vi "synchronization_0.vi"(11 "sweep signal":dbl[](array[numeric])=array[10000 elements]) -> (0 "Micro 1/ ai 2":dbl[](graph), 3 "Micro 2/ai 1":dbl[](graph))   [LabVIEW 2014]
uses:
  <vilib>/DAQmx/configure/timing.llb/DAQmx Timing (Sample Clock).vi
  <vilib>/DAQmx/create/channels.llb/DAQmx Create Channel (AO-Voltage-Basic).vi
  <vilib>/DAQmx/write.llb/DAQmx Write (Analog 1D DBL 1Chan NSamp).vi
  <vilib>/DAQmx/create/channels.llb/DAQmx Create Channel (AI-Voltage-Basic).vi
  <vilib>/DAQmx/read.llb/DAQmx Read (Analog 2D DBL NChan NSamp).vi
panel:
  out "Sweep":dbl[](graph)
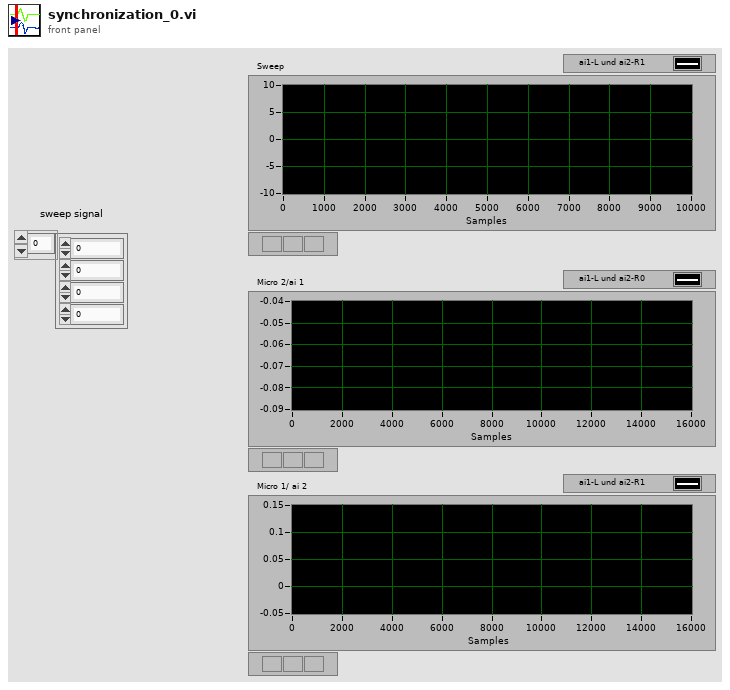
[diagram p1: front panel]
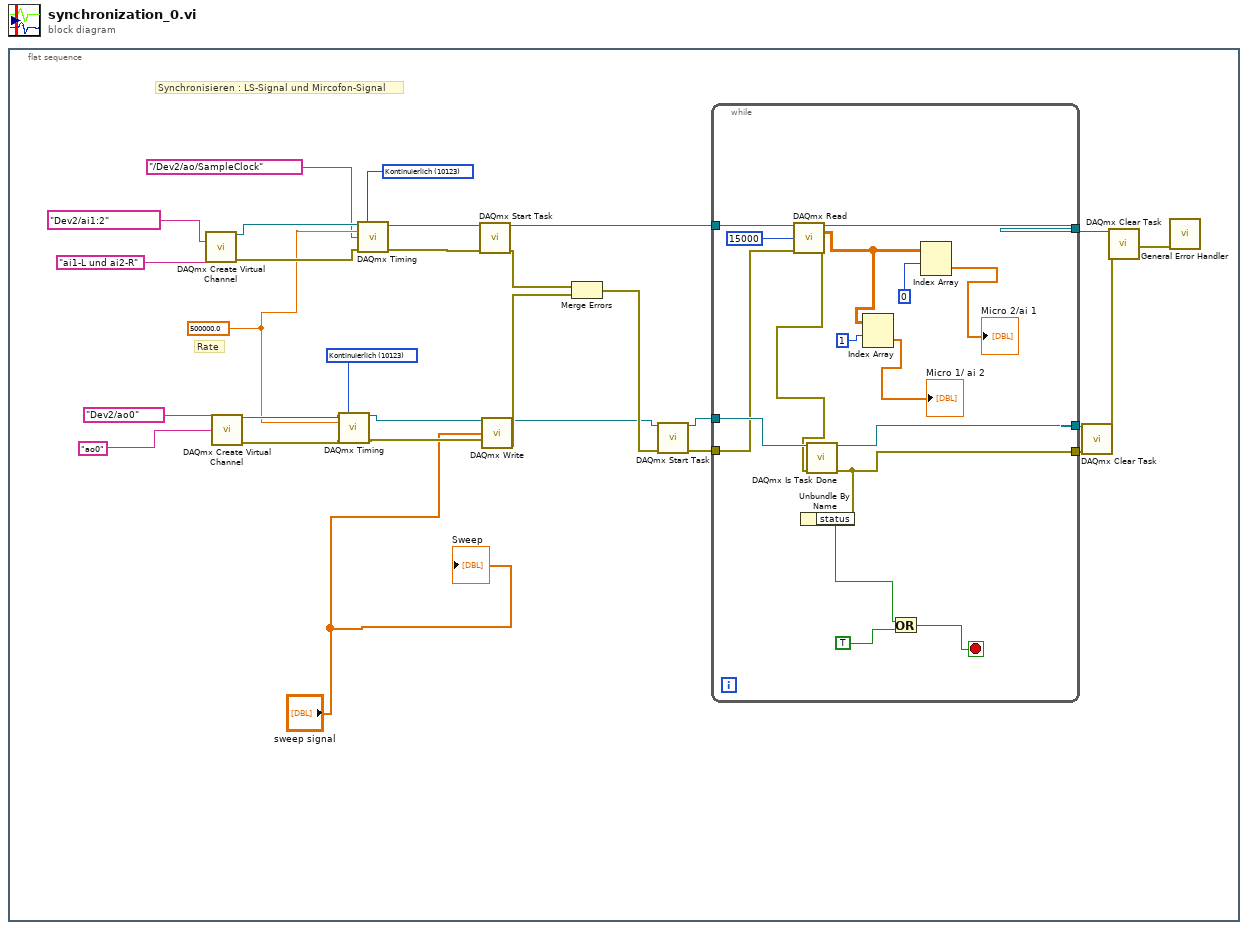
[diagram p0: block diagram]
diagram:
  n1 = flat-sequence {
    frame #0 {
      w5 = 10123 items=["Endliche Anzahl"=10178, "Kontinuierlich"=10123, "Einzelwert (HW-getaktet)"=12522] ("sample mode")
      w8 = 500000.0 ("rate")
      w23 = 10123 items=["Endliche Anzahl"=10178, "Kontinuierlich"=10123, "Einzelwert (HW-getaktet)"=12522] ("sample mode")
      # "Synchronisieren : LS-Signal und Mircofon-Signal"
      # "Rate"
      n2 = call-poly <vilib>:"DAQmx Create Virtual Channel.vi"("physical channels"=tag "Dev2/ai1:2" ("physical channels 2"), "name to assign"="ai1-L und ai2-R") -> ("task out"=w18:refnum<k21>, "error out"=w29:errorcluster)  [unwired: 12 in]
      n3 = call-poly <vilib>:"DAQmx Create Virtual Channel.vi"("physical channels"=tag "Dev2/ao0", "name to assign"="ao0") -> ("task out"=w27:refnum<k21>, "error out"=w24:errorcluster)  [unwired: 12 in]
      n4 = call-poly <vilib>:"DAQmx Timing.vi"("task/channels in"=w27, "sample mode"=w23, "rate"=w8, "error in"=w24) -> ("task out"=w26:refnum<k21>, "error out"=w25:errorcluster)  [unwired: 10 in]
      n5 = call-poly <vilib>:"DAQmx Timing.vi"("task/channels in"=w18, "sample mode"=w5, "rate"=w8, "source"=tag "/Dev2/ao/SampleClock", "error in"=w29) -> ("task out"=w22:refnum<k21>, "error out"=w9:errorcluster)  [unwired: 9 in]
      n6 = call <vilib>:"DAQmx Start Task.vi"("task/channels in"=w22, "error in"=w9) -> ("task out"=w13:refnum<k21>, "error out"=w20:errorcluster)  [unwired: 12 in]
      n7 = call-poly <vilib>:"DAQmx Write.vi"("task/channels in"=w26, "data"="sweep signal", "error in"=w25) -> ("task out"=w6:refnum<k21>, "error out"=w7:errorcluster)  [unwired: 10 in, 1 out]
      n8 = Merge Errors(w20, w7) -> (w19:errorcluster)
      n9 = call <vilib>:"DAQmx Start Task.vi"("task/channels in"=w6, "error in"=w19) -> ("task out"=w3:refnum<k21>, "error out"=w2:errorcluster)  [unwired: 12 in]
      n10 = while {
        tunnel: [w35] -> w14
        tunnel: w13 -> [w38]
        tunnel: w2 -> [w37]
        tunnel: w3 -> [w45]
        tunnel: [w44] -> w12
        tunnel: [w41] -> w11
        stop <- w43 stop-if-true
        n11 = call-poly <vilib>:"DAQmx Read.vi"("task/channels in"=w38, "number of samples per channel"=15000, "error in"=w37) -> ("task out"=w35:refnum<k21>, "data"=w30:dbl[][], "error out"=w36:errorcluster)  [unwired: 10 in]
        n12 = call <vilib>:"DAQmx Is Task Done.vi"("task/channels in"=w45, "error in"=w36) -> ("task out"=w44:refnum<k21>, "error out"=w41:errorcluster)  [unwired: 11 in, 1 out]
        n13 = Unbundle By Name(w41) -> ("status"=w40:bool)
        n14 = Index Array(array=w30, index (row)=1 ("Index")) -> (element=→"Micro 1/ ai 2":dbl[])  [unwired: 1 in]
        n15 = Or(x=w40, y=TRUE) -> (x .or. y?=w43:bool)
        n16 = Index Array(array=w30, index (row)=0 ("Index")) -> (element=→"Micro 2/ai 1":dbl[])  [unwired: 1 in]
      }
      n17 = call <vilib>:"DAQmx Clear Task.vi"("task in"=w12, "error in"=w11) -> ("error out"=w10:errorcluster)  [unwired: 13 in]
      n18 = call <vilib>:"DAQmx Clear Task.vi"("task in"=w14, "error in"=w10) -> ("error out"=w28:errorcluster)  [unwired: 13 in]
      n19 = call <vilib>:"General Error Handler.vi"("error in (no error)"=w28) -> ()  [unwired: 10 in, 5 out]
      "Sweep" <- "sweep signal"
    }
  }
